vi "absortion_comparation.vi"() -> ()   [LabVIEW 2021]
uses:
  <vilib>/Utility/file.llb/Read Delimited Spreadsheet (DBL).vi
panel:
  out "Muestra 2":cluster{"all rows":dbl[], "all rows":dbl[]}(graph)={"all rows"=[0.001, 0.0015, 0.002, 0.003, 0.004, 0.005, 0.006, 0.008, 0.01, 0.015, 0.02, 0.03, 0.04, 0.05, 0.06, 0.08, 0.1, 0.15, 0.2, 0.3, 0.4, 0.5, 0.6, 0.8, 1.0, 1.25, 1.5, 2.0, 3.0, 4.0, 5.0, 6.0, 8.0, 10.0, 15.0, 20.0], "all rows"=[4078.0, 1376.0, 617.3, 192.9, 82.78, 42.58, 24.64, 10.37, 5.329, 1.673, 0.8096, 0.3756, 0.2683, 0.2269, 0.2059, 0.1837, 0.1707, 0.1505, 0.137, 0.1186, 0.1061, 0.09687, 0.08956, 0.07865, 0.07072, 0.06323, 0.05754, 0.04942, 0.03969, 0.03403, 0.03031, 0.0277, 0.02429, 0.02219, 0.01941, 0.01813]}
  out "Comparación de coeficientes de absorción":cluster{"Energia":dbl[], "coeficiente":dbl[]}[](graph)
  in  "Muestra 2":path=path "C:/Users/pbellido/Desktop/TEMAS PR_ALARA/COEFICIENTS_DATA/WATER.txt"
  in  "error in (no error) 2":errorcluster
  out "Muestra 1":cluster{"all rows":dbl[], "all rows":dbl[]}(graph)={"all rows"=[0.001, 0.0015, 0.002, 0.003, 0.004, 0.005, 0.006, 0.008, 0.01, 0.015, 0.02, 0.03, 0.04, 0.05, 0.06, 0.08, 0.1, 0.15, 0.2, 0.3, 0.4, 0.5, 0.6, 0.8, 1.0, 1.25, 1.5, 2.0, 3.0, 4.0, 5.0, 6.0, 8.0, 10.0, 15.0, 20.0], "all rows"=[4078.0, 1376.0, 617.3, 192.9, 82.78, 42.58, 24.64, 10.37, 5.329, 1.673, 0.8096, 0.3756, 0.2683, 0.2269, 0.2059, 0.1837, 0.1707, 0.1505, 0.137, 0.1186, 0.1061, 0.09687, 0.08956, 0.07865, 0.07072, 0.06323, 0.05754, 0.04942, 0.03969, 0.03403, 0.03031, 0.0277, 0.02429, 0.02219, 0.01941, 0.01813]}
  in  "error in (no error)":errorcluster
  in  "Muestra 1":path=path "C:/Users/pbellido/Desktop/TEMAS PR_ALARA/COEFICIENTS_DATA/WATER.txt"
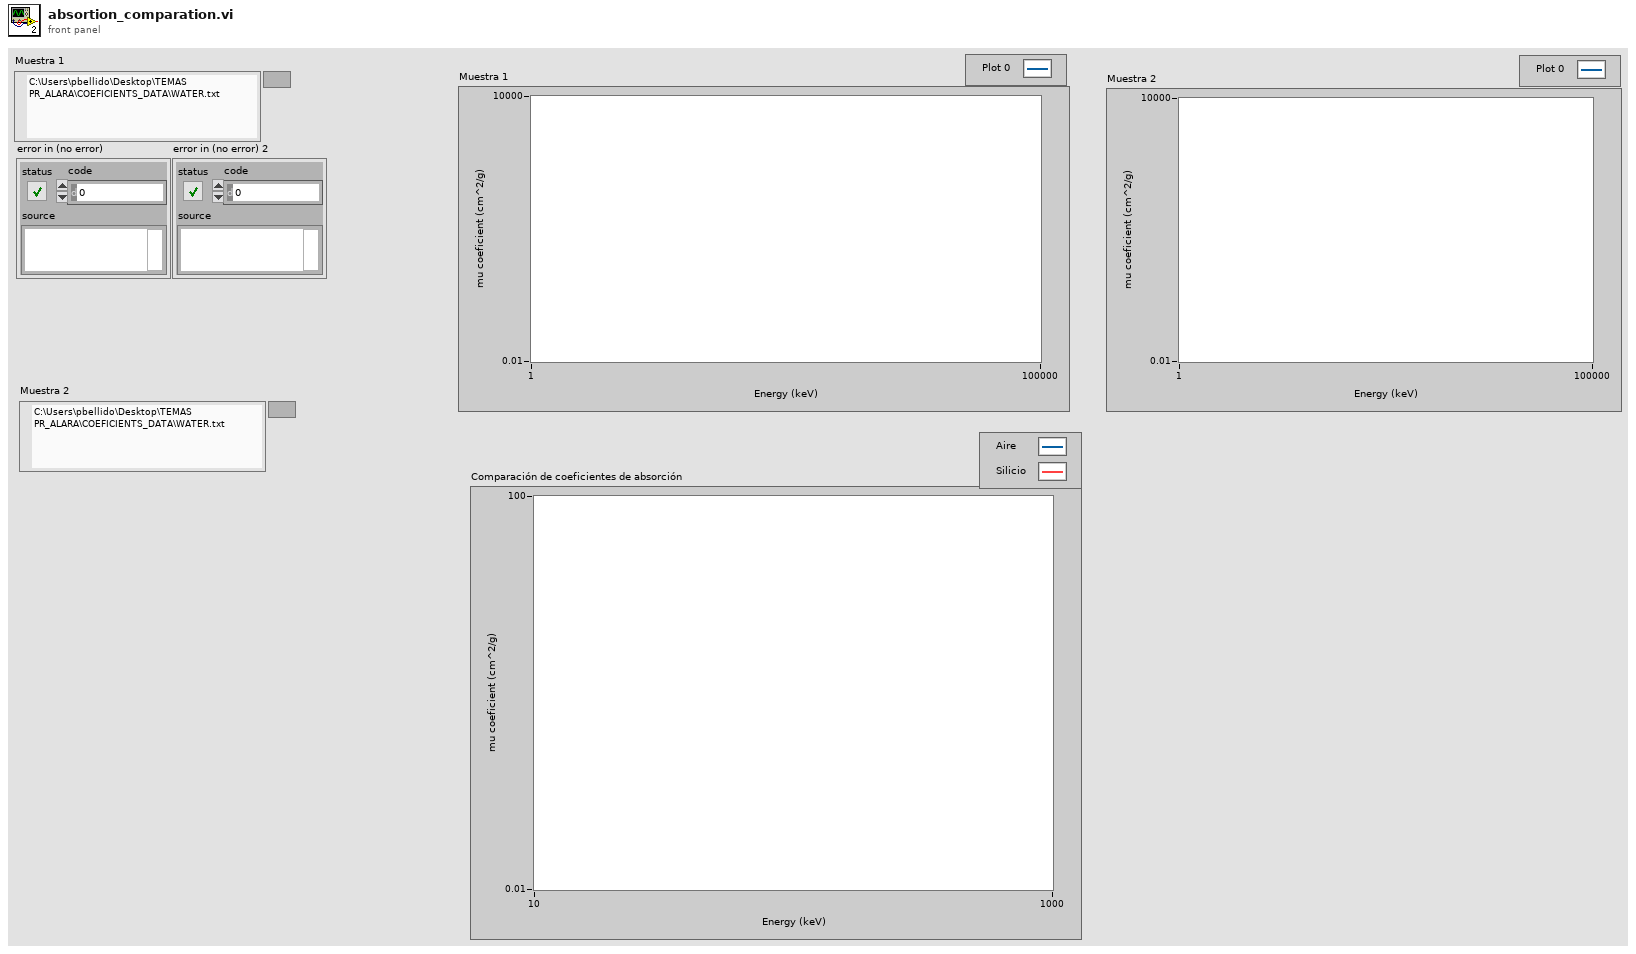
[diagram p1: front panel]
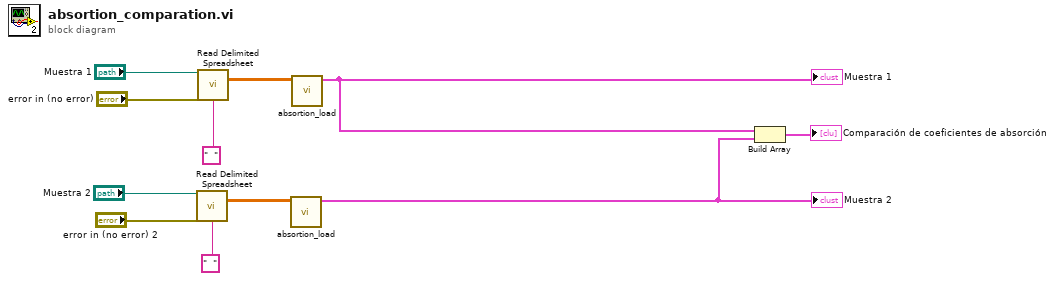
[diagram p0: block diagram]
diagram:
  n1 = call-poly <vilib>:"Read Delimited Spreadsheet.vi"("file path (dialog if empty)"="Muestra 2", "error in (no error)"="error in (no error) 2", "delimiter (\\t)"="  " ("delimiter (\\t)")) -> ("all rows"=w7:dbl[][])  [unwired: 7 in, 5 out]
  n2 = call-poly <vilib>:"Read Delimited Spreadsheet.vi"("file path (dialog if empty)"="Muestra 1", "error in (no error)"="error in (no error)", "delimiter (\\t)"="  " ("delimiter (\\t)")) -> ("all rows"=w8:dbl[][])  [unwired: 7 in, 5 out]
  n3 = call "absortion_load.vi"("all rows"=w7) -> ("curva atenuation"=w1:cluster{"Energia":dbl[], "coeficiente":dbl[]})  [unwired: 10 in]
  "Muestra 2" <- w1
  n4 = call "absortion_load.vi"("all rows"=w8) -> ("curva atenuation"=w3:cluster{"Energia":dbl[], "coeficiente":dbl[]})  [unwired: 10 in]
  "Muestra 1" <- w3
  n5 = Build Array(w3, w1) -> (→"Comparación de coeficientes de absorción":cluster{"Energia":dbl[], "coeficiente":dbl[]}[])
